vi "XML ( Set Node Value Single Input ).vi"(8 "error in (no error)":errorcluster, 9 "Value":string, 10 "XPath expression":string, 11 "XML in":refnum<class "XML.lvclass">) -> (0 "error out":errorcluster, 3 "XML out":refnum<class "XML.lvclass">)   [LabVIEW 2018, in "XML.lvlib" / "XML.lvclass"]
uses:
  XML.lvclass
  XML.lvclass/XML.ctl
  <vilib>/xml/NI_XML.lvlib
  <resource>/objmgr/DOMUserDefRef.rc
  <vilib>/xml/Close Reference(Node).vi
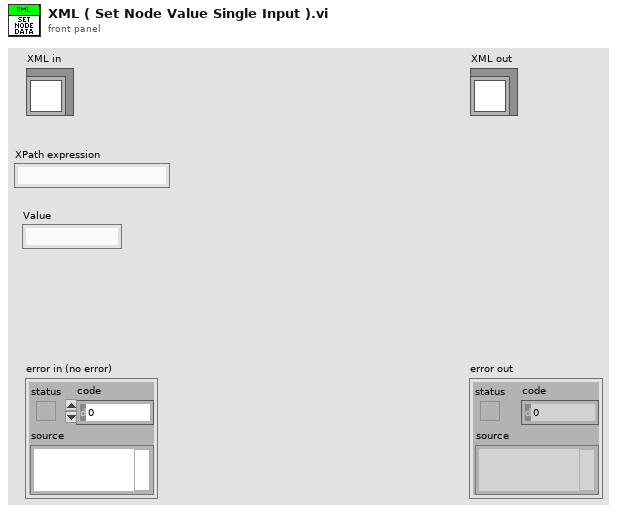
[diagram p1: front panel]
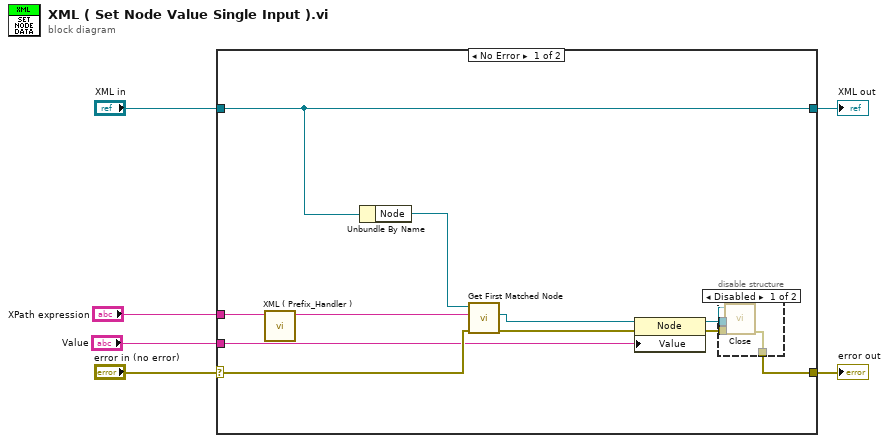
[diagram p0: block diagram]
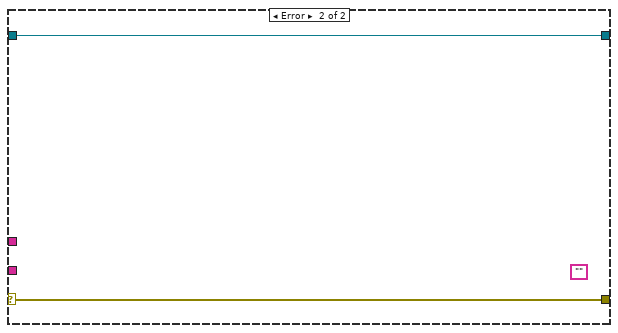
[diagram p3: hidden frame]
diagram:
  n1 = case shown="No Error" "error in (no error)" {
    selector: "error in (no error)" -> [w15 w22]
    tunnel: [w12 w22] -> w5
    tunnel: [w17 w21] -> w3
    tunnel: "XML in" -> [w17 w21]
    tunnel: "XPath expression" -> [w11 _]
    tunnel: "Value" -> [w9 _]
    frame No Error {
      n2 = call "XML ( Prefix_Handler ).vi"("input string"=w11) -> ("result string"=w10:string)  [unwired: 10 in]
      n3 = Unbundle By Name(w17) -> ("Node"=w16:refnum<k20>)
      n4 = call <vilib>:"Get First Matched Node.vi"("error in (no error)"=w15, "XPath expression"=w10, "node in"=w16) -> ("error out"=w7:errorcluster, "node result"=w8:refnum<k20>)  [unwired: 6 in, 1 out]
      n5 = property class="Node"(reference=w8, error in=w7, "Value"=w9) -> (reference out=w13:refnum<k20>, error out=w14:errorcluster)
      n6 = disable-structure shown="Disabled" {
        disable-tunnel: w14 -> [w20 _]
        disable-tunnel: w13 -> [w19 _]
        disable-tunnel: [w18 _] -> w12
        frame Disabled {
          n7 = call-poly <vilib>:"Close.vi"("error in (no error)"=w20, "node"=w19) -> ("error out"=w18:errorcluster)  [unwired: 7 in]
        }
        frame Enabled {
        }
      }
    }
    frame Error {
      (unwired) ""
    }
  }
  "error out" <- w5
  "XML out" <- w3
